vi "Load.vi"(8 "error in (no error)":errorcluster) -> (0 "error out":errorcluster)   [LabVIEW 2021, in "Markdown.lvlib"]
doc: "Load the library project references."
uses:
  Markdown.lvlib
  TypeDefs/Item.ctl
  Global.vi
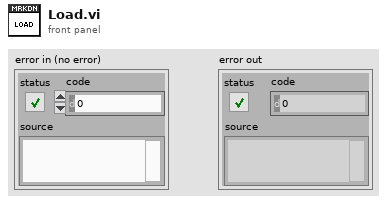
[diagram p1: front panel]
types:
  T1 = typedef "Markdown.lvlib/Item.ctl" = cluster{"Name":string, "Icon":picture, "Path":path, "Title":string, "Desc":string, "ConPane":picture, "TypeString":string, "ProjectItem":string, "VI Type":enum32{"invalid VI type", "Standard VI", "Control VI", "Global VI", "Polymorphic VI", "Configuration VI", "SubSystem", "Facade VI", "Method VI", "Statechart Diagram VI"}}
  T2 = enum32{"invalid VI type", "Standard VI", "Control VI", "Global VI", "Polymorphic VI", "Configuration VI", "SubSystem", "Facade VI", "Method VI", "Statechart Diagram VI"}
  T3 = typedef "imagedata.ctl" = cluster{"image type":i32, "image depth":i32, "image":u8[], "mask":u8[], "colors":u32[], "Rectangle":cluster{"left":i16, "top":i16, "right":i16, "bottom":i16}}
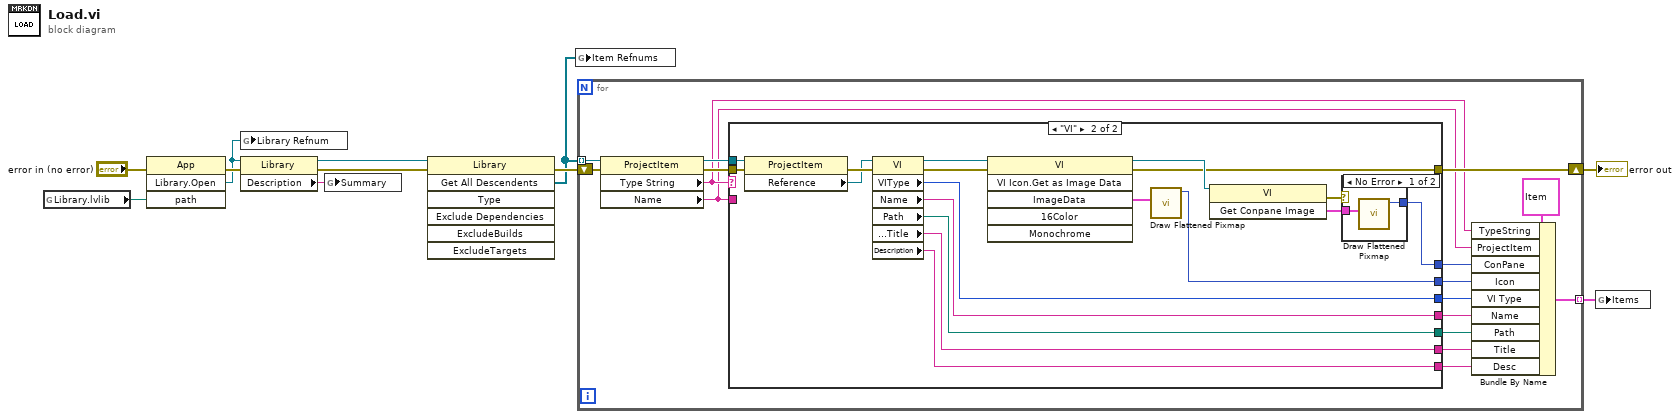
[diagram p0: block diagram]
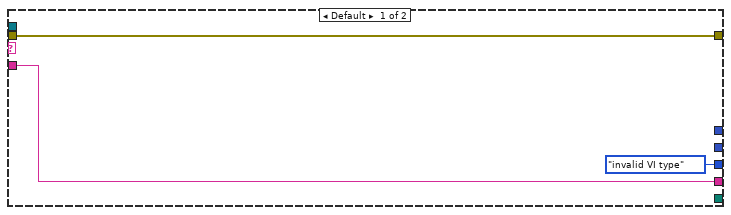
[diagram p2: hidden frame]
diagram:
  n1 = global read "Global.vi" "Library.lvlib"() -> (w5:path)
  n2 = invoke class="App" method="Library.Open"(error in="error in (no error)", "path"=w5) -> (error out=w11:errorcluster, "Open Library"=w4:refnum<vi>)  [unwired: 2 in, 2 out]
  n3 = global write "Global.vi" "Library Refnum"(w4) -> ()
  n4 = property class="Library"(reference=w4, error in=w11) -> (reference out=w7:refnum<vi>, error out=w8:errorcluster, "Description"=w3:string)
  n5 = global write "Global.vi" "Summary"(w3) -> ()
  n6 = invoke class="Library" method="Get All Descendents"(reference=w7, error in=w8) -> (error out=w6:errorcluster, "All Descendents"=w2:refnum<vi>[])  [unwired: 5 in, 5 out]
  n7 = global write "Global.vi" "Item Refnums"(w2) -> ()
  n8 = for {
    tunnel: w2 -> [w26] mode=indexing
    shift-right: [w24] -> w9
    shift-left: w6 -> [w27]
    tunnel: [w16] -> w1 mode=indexing
    n9 = property class="ProjectItem"(reference=w26, error in=w27) -> (reference out=w23:refnum<vi>, error out=w25:errorcluster, "Type String"=w14:string, "Name"=w13:string)
    n10 = case shown="\"VI\"" w14 {
      tunnel: w25 -> [w30 w48]
      tunnel: [w30 w38] -> w24
      tunnel: w23 -> [_ w46]
      tunnel: w13 -> [w29 _]
      tunnel: [_ w37] -> w21
      tunnel: [w29 w36] -> w20
      tunnel: [_ w35] -> w19
      tunnel: [_ w34] -> w18
      tunnel: [_ w33] -> w17
      tunnel: [_ w32] -> w15
      tunnel: [T2."invalid VI type" ("VIType") w31] -> w12
      frame Default {
      }
      frame "VI" {
        n11 = property class="ProjectItem"(reference=w46, error in=w48) -> (error out=w47:errorcluster, "Reference"=w44:refnum<vi>)  [unwired: 1 out]
        n12 = property class="VI"(reference=w44, error in=w47) -> (reference out=w43:refnum<vi>, error out=w45:errorcluster, "VIType"=w31:T2, "Name"=w36:string, "Path"=w35:path, "Front Panel.Title"=w34:string, "Description"=w33:string)
        n13 = invoke class="VI" method="VI Icon.Get as Image Data"(reference=w43, error in=w45) -> (reference out=w41:refnum<vi>, error out=w38:errorcluster, "ImageData"=w42:T3)  [unwired: 4 in, 3 out]
        n14 = call <vilib>:"Draw Flattened Pixmap.vi"("image data"=w42) -> ("new picture"=w37:picture)  [unwired: 8 in]
        n15 = invoke class="VI" method="Get Conpane Image"(reference=w41) -> (error out=w39:errorcluster, "Get Conpane Image"=w40:T3)  [unwired: 2 in, 1 out]
        n16 = case shown="No Error" w39 {
          tunnel: w40 -> [w50 _]
          tunnel: [w49 _] -> w32
          frame No Error {
            n17 = call <vilib>:"Draw Flattened Pixmap.vi"("image data"=w50) -> ("new picture"=w49:picture)  [unwired: 8 in]
          }
          frame Error {
          }
        }
      }
    }
    n18 = Bundle By Name(cluster=T1 {"Name"="", "Icon"=bytes[0], "Path"=path "", "Title"="", "Desc"="", "ConPane"=bytes[0], "TypeString"="", "ProjectItem"="", "VI Type"=enum."invalid VI type"} ("Item"), "TypeString"=w14, "ProjectItem"=w13, "ConPane"=w15, "Icon"=w21, "VI Type"=w12, "Name"=w20, "Path"=w19, "Title"=w18, "Desc"=w17) -> (w16:T1)
  }
  "error out" <- w9
  n19 = global write "Global.vi" "Items"(w1) -> ()
